vi "headingoperater.vi"(9 "h1":dbl, 11 "h2":dbl) -> (2 "h2-h1":dbl, 3 "h2+h1":dbl)   [LabVIEW 2015]
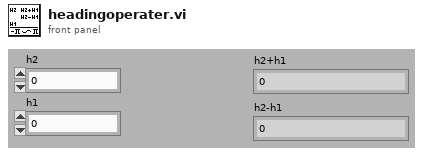
[diagram p1: front panel]
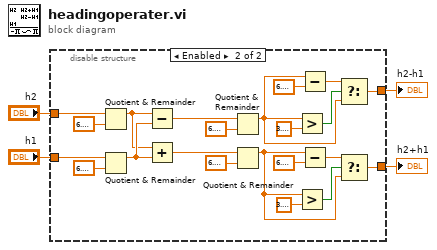
[diagram p0: block diagram]
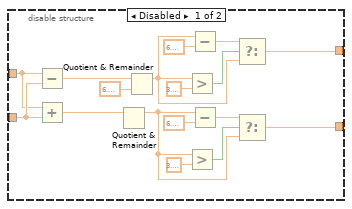
[diagram p2: hidden frame]
diagram:
  n1 = disable-structure shown="Enabled" {
    disable-tunnel: [w20 w24] -> w1
    disable-tunnel: [w7 w32] -> w2
    disable-tunnel: "h1" -> [w6 w40]
    disable-tunnel: "h2" -> [w5 w42]
    frame Disabled {
      n2 = Subtract(x=w5, y=w6) -> (x-y=w21:dbl)
      n3 = Add(x=w5, y=w6) -> (x+y=w8:dbl)
      n4 = Quotient & Remainder(x=w8) -> (x-y*floor(x/y)=w13:dbl)  [unwired: 1 in, 1 out]
      n5 = Quotient & Remainder(x=w21, y=6.283185307179586) -> (x-y*floor(x/y)=w14:dbl)  [unwired: 1 out]
      n6 = Greater?(x=w14, y=3.141592653589793) -> (0:w17:bool)
      n7 = Greater?(x=w13, y=3.141592653589793) -> (0:w10:bool)
      n8 = Subtract(x=w14, y=6.283185307179586) -> (x-y=w16:dbl)
      n9 = Subtract(x=w13, y=6.283185307179586) -> (x-y=w11:dbl)
      n10 = Select(t=w16, s=w17, f=w14) -> (s? t:f=w20:dbl)
      n11 = Select(t=w11, s=w10, f=w13) -> (s? t:f=w7:dbl)
    }
    frame Enabled {
      n12 = Quotient & Remainder(x=w42, y=6.283185307179586) -> (x-y*floor(x/y)=w22:dbl)  [unwired: 1 out]
      n13 = Quotient & Remainder(x=w40, y=6.283185307179586) -> (x-y*floor(x/y)=w23:dbl)  [unwired: 1 out]
      n14 = Subtract(x=w22, y=w23) -> (x-y=w25:dbl)
      n15 = Add(x=w22, y=w23) -> (x+y=w33:dbl)
      n16 = Quotient & Remainder(x=w25, y=6.283185307179586) -> (x-y*floor(x/y)=w26:dbl)  [unwired: 1 out]
      n17 = Quotient & Remainder(x=w33, y=6.283185307179586) -> (x-y*floor(x/y)=w39:dbl)  [unwired: 1 out]
      n18 = Greater?(x=w26, y=3.141592653589793) -> (0:w29:bool)
      n19 = Greater?(x=w39, y=3.141592653589793) -> (0:w36:bool)
      n20 = Subtract(x=w26, y=6.283185307179586) -> (x-y=w28:dbl)
      n21 = Subtract(x=w39, y=6.283185307179586) -> (x-y=w37:dbl)
      n22 = Select(t=w28, s=w29, f=w26) -> (s? t:f=w24:dbl)
      n23 = Select(t=w37, s=w36, f=w39) -> (s? t:f=w32:dbl)
    }
  }
  "h2+h1" <- w2
  "h2-h1" <- w1
